vi "odometryfgv.vi"(7 "error in (no error)":errorcluster, 9 "wheelbase":dbl=250.0, 10 "Reset":bool) -> (0 "error out":errorcluster, 2 "XY Graph 2":cluster{"X":dbl, "Y":dbl}[](graph), 3 "X, Y, BEARING":cluster{dbl, dbl, dbl}={77.90712658947966, 981.2627307621673, -194.46797875856427})   [LabVIEW 2017]
uses:
  <vilib>/myRIO/Common/Instrument Driver Framework/myRIO v1.0/Encoder/typedefs/Encoder Signal Mode.ctl
  <vilib>/myRIO/Instrument Drivers/Onboard IO/Encoder/typedefs/Encoder Reference.ctl
  <vilib>/myRIO/Common/Instrument Driver Framework/Utilities/typedefs/myRIO Generic Hardware Reference.ctl
  <vilib>/myRIO/Common/Instrument Driver Framework/Utilities/typedefs/Hardware Version Enum.ctl
  <vilib>/myRIO/Common/Instrument Driver Framework/Utilities/typedefs/myRIO v1.0 Reference.ctl
  <vilib>/myRIO/Common/Instrument Driver Framework/Utilities/typedefs/Generic FPGA Reference.ctl
  <vilib>/myRIO/Common/Instrument Driver Framework/myRIO v1.0/Encoder/typedefs/Encoder Channels Enum.ctl
  <vilib>/myRIO/Common/Instrument Driver Framework/myRIO v1.0/Encoder/typedefs/Encoder Configuration v1.0.ctl
  <vilib>/userdefined/High Color/nirio_resource_hc.ctl
  <vilib>/myRIO/Common/Instrument Driver Framework/Utilities/vis/Is FPGA Ref Available.vi
  <vilib>/myRIO/Common/Instrument Driver Framework/myRIO v1.0/Encoder/vis/myRIO v1.1 Open Encoder.vi
  <vilib>/myRIO/Instrument Drivers/Onboard IO/Encoder/vis/Read.vi
  <vilib>/myRIO/Common/Instrument Driver Framework/Utilities/vis/Validate Channels.vi
  <vilib>/myRIO/Common/Instrument Driver Framework/myRIO v1.0/Encoder/vis/myRIO v1.0 Reserve Encoder.vi
  <vilib>/myRIO/Common/Instrument Driver Framework/myRIO v1.0/Encoder/vis/myRIO v1.0 Build MUX Configuration Encoder.vi
  <vilib>/myRIO/Common/Instrument Driver Framework/myRIO v1.0/Resource Manager/vis/myRIO v1.0 Reserve Channel List.vi
  <vilib>/myRIO/Common/Instrument Driver Framework/myRIO v1.0/Resource Manager/vis/myRIO v1.0 Create Configuration List.vi
  <vilib>/myRIO/Common/Instrument Driver Framework/myRIO v1.0/Resource Manager/vis/myRIO v1.0 Reserve Channel.vi
  <vilib>/myRIO/Common/Instrument Driver Framework/myRIO v1.0/Resource Manager/vis/myRIO v1.0 Unreserve Channel.vi
  <vilib>/myRIO/Common/Instrument Driver Framework/myRIO v1.0/Resource Manager/vis/myRIO v1.0 Build Mutex Name.vi
  <vilib>/Utility/VariantDataType/GetNumericInfo.vi
  <vilib>/Utility/error.llb/Error Cluster From Error Code.vi
  <vilib>/myRIO/Common/Instrument Driver Framework/myRIO v1.0/myRIO v1.1 Open.vi
  <vilib>/myRIO/Common/Instrument Driver Framework/Utilities/vis/IO Manager.vi
  <vilib>/myRIO/Common/Instrument Driver Framework/Utilities/vis/Configuration Manager.vi
  <vilib>/myRIO/Common/Instrument Driver Framework/myRIO v1.0/Resource Manager/vis/myRIO v1.0 Configure IO.vi
  <vilib>/myRIO/Common/Instrument Driver Framework/myRIO v1.0/myRIO v1.0 Close.vi
  <vilib>/myRIO/Common/Instrument Driver Framework/myRIO v1.0/Encoder/vis/myRIO v1.0 Configure Encoder.vi
  <vilib>/myRIO/Common/Instrument Driver Framework/myRIO v1.0/Encoder/vis/myRIO v1.0 Read Encoder.vi
  <vilib>/myRIO/Express VI/Onboard IO/Encoder/Encoder Express VI.xnode
  <vilib>/myRIO/Instrument Drivers/Onboard IO/Encoder/vis/myRIO Encoder Open.xnode
  <vilib>/myRIO/Instrument Drivers/Onboard IO/Encoder/Encoder.lvlib
panel:
  out "Waveform Chart":cluster{dbl, dbl, dbl}(graph)
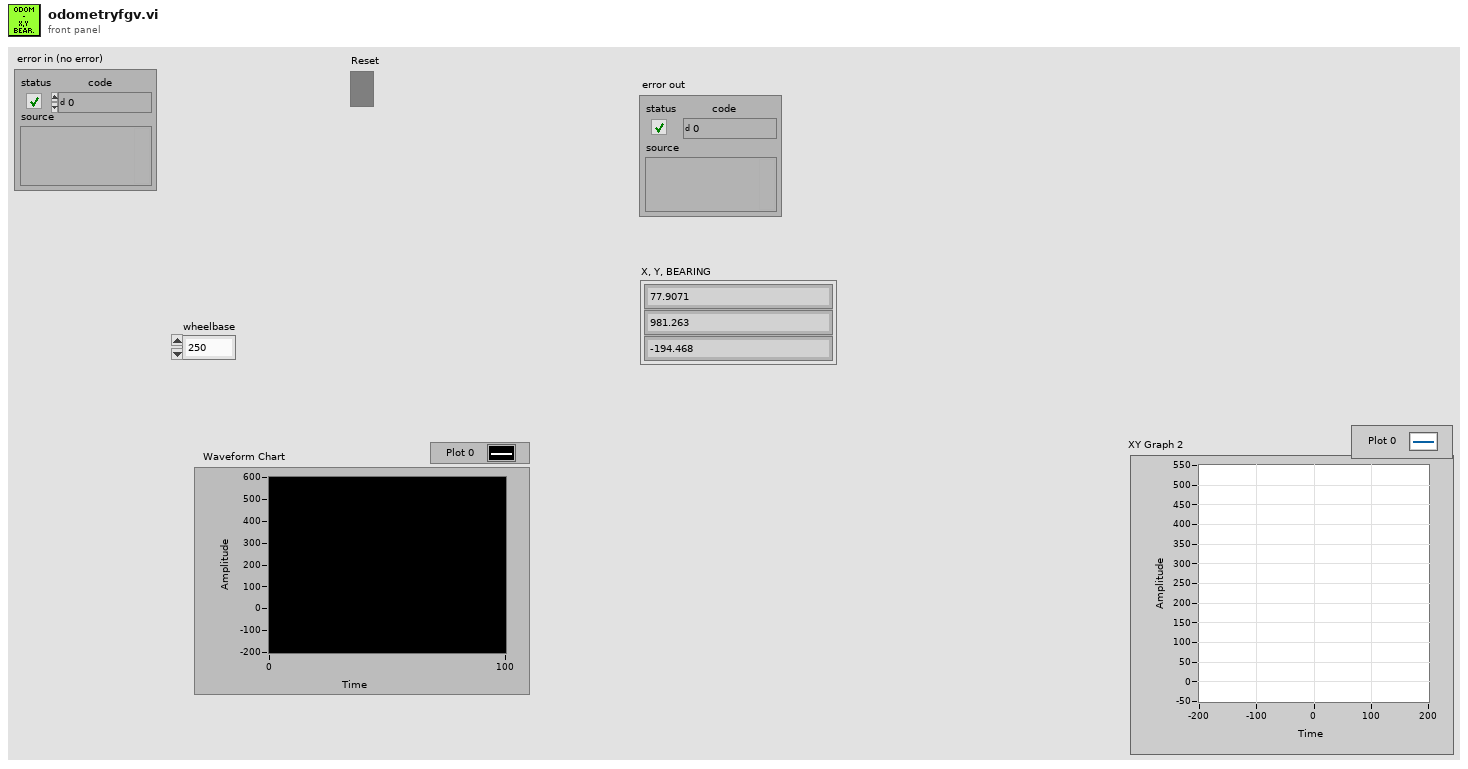
[diagram p1: front panel]
types:
  T1 = typedef "Encoder.lvlib/Encoder Reference.ctl" = cluster{"myRIO Reference":T2, "Encoder Channels Enum":T6}
  T2 = typedef "myRIO Generic Hardware Reference.ctl" = cluster{"myRIO Model":T3, "myRIO Hardware Reference":T4}
  T3 = typedef "Hardware Version Enum.ctl" = enum16{"Unknown", "myRIO-1900", "myRIO-1950", "roboRIO", "NI ELVIS RIO CM"}
  T4 = typedef "myRIO v1.0 Reference.ctl" = cluster{"Generic FPGA Reference":T5, "Allow multiple opens":bool}
  T5 = typedef "Generic FPGA Reference.ctl" = refnum<k20>
  T6 = typedef "Encoder Channels Enum.ctl" = enum16{"Not Connected", "C/ENC0", "C/ENC1", "A/ENC", "B/ENC", "DIO/ENC0", "DIO/ENC1", "DIO/ENC2", "DIO/ENC3", "DIO/ENC4"}
  T7 = typedef "Encoder Signal Mode.ctl" = enum16{"Quadrature phase signal", "Step and direction signal"}
  T8 = typedef "nirio_resource_hc.ctl" = tag
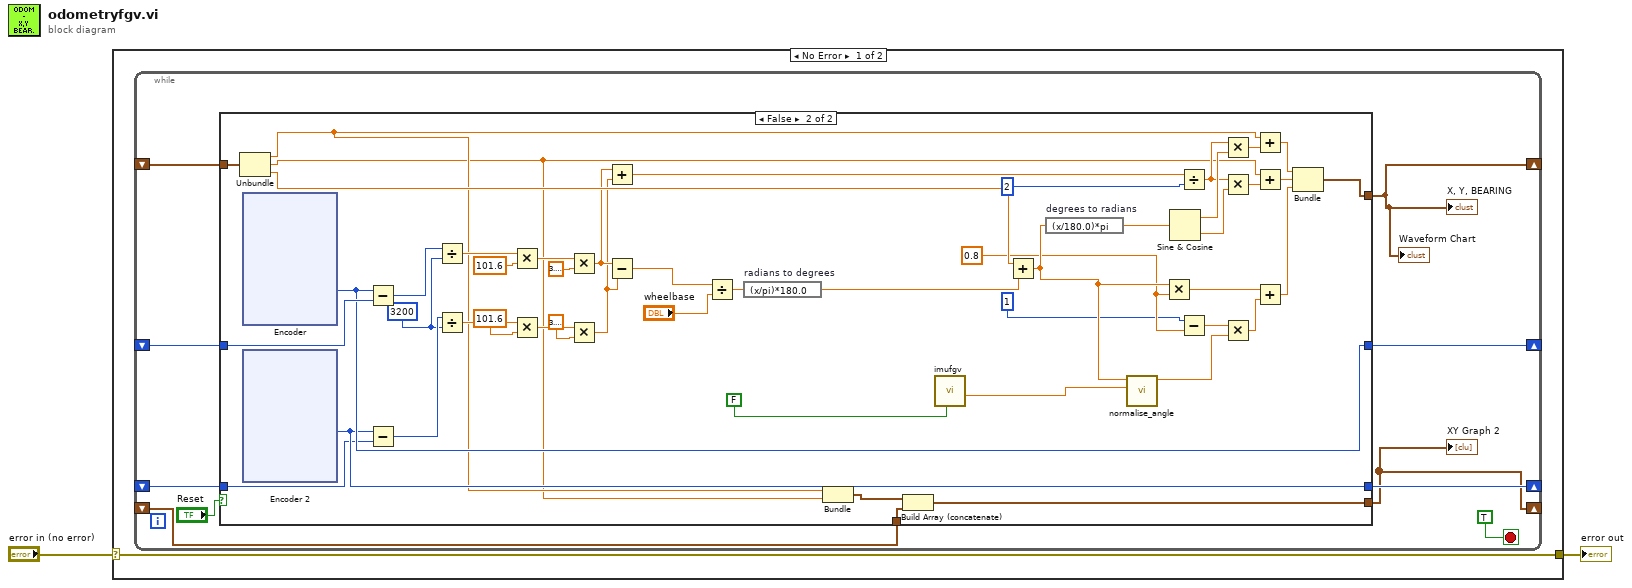
[diagram p0: block diagram]
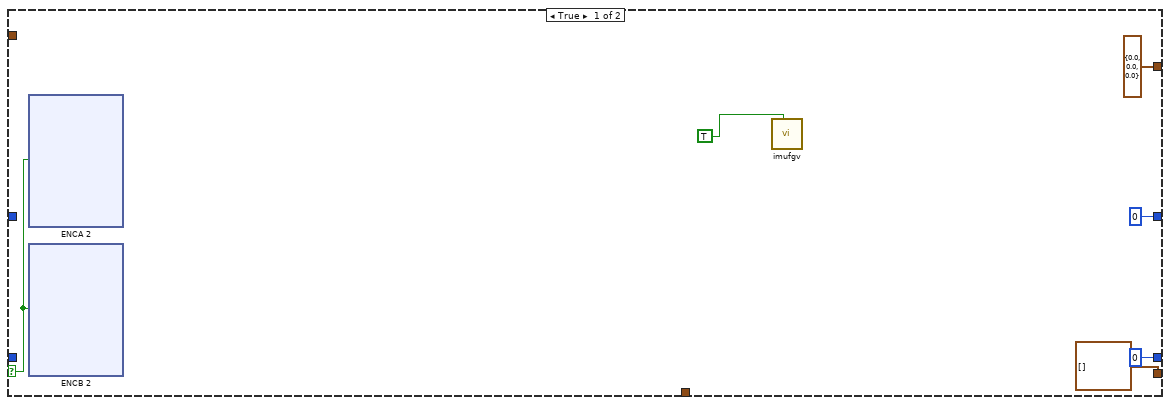
[diagram p2: hidden frame]
diagram:
  n1 = case shown="No Error" "error in (no error)" {
    selector: "error in (no error)" -> [w3 w253]
    tunnel: [w3 w253] -> w1
    frame No Error {
      n2 = while {
        shift-right: [w6] -> _
        shift-left: _ -> [w13]
        shift-right: [w11] -> _
        shift-left: _ -> [w10]
        shift-right: [w9] -> _
        shift-left: _ -> [w8]
        shift-right: [w4] -> _
        shift-left: _ -> [w5]
        stop <- TRUE stop-if-true
        n3 = case shown="False" "Reset" {
          selector: "Reset" -> [w16 _]
          tunnel: w13 -> [_ w160]
          tunnel: [cluster{dbl, dbl, dbl} {0.0, 0.0, 0.0} w118] -> w6
          tunnel: w10 -> [_ w149]
          tunnel: [0 w131] -> w11
          tunnel: [0 w130] -> w9
          tunnel: w8 -> [_ w129]
          tunnel: [cluster{dbl, dbl}[] [] w113] -> w4
          tunnel: w5 -> [_ w112]
          frame True {
            n4 = xnode "ENCA 2"("Reset Counter"=w16) -> ()  [unwired: 1 in, 4 out]
            n5 = xnode "ENCB 2"("Reset Counter"=w16) -> ()  [unwired: 1 in, 4 out]
            n6 = call "imufgv.vi"("Rset"=TRUE) -> ()  [unwired: 9 in, 2 out]
          }
          frame False {
            w122 = 0.8
            w144 = 3200
            n7 = Unbundle(w160) -> (w116:dbl, w115:dbl, w156:dbl)
            n8 = xnode "Encoder"() -> ("Counter Value"=w131:i32)  [unwired: 2 in, 3 out]
            n9 = xnode "Encoder 2"() -> ("Counter Value"=w130:i32)  [unwired: 2 in, 3 out]
            n10 = Subtract(x=w131, y=w149) -> (x-y=w146:i32)
            n11 = Subtract(x=w130, y=w129) -> (x-y=w145:i32)
            n12 = Divide(x=w146, y=w144) -> (x/y=w143:dbl)
            n13 = Divide(x=w145, y=w144) -> (x/y=w135:dbl)
            n14 = Multiply(x=w143, y=101.6) -> (x*y=w142:dbl)
            n15 = Multiply(x=w135, y=101.6) -> (x*y=w137:dbl)
            n16 = Multiply(x=w142, y=3.141592653589793) -> (x*y=w141:dbl)
            n17 = Multiply(x=w137, y=3.141592653589793) -> (x*y=w136:dbl)
            n18 = Add(x=w141, y=w136) -> (x+y=w147:dbl)
            n19 = Subtract(x=w141, y=w136) -> (x-y=w148:dbl)
            n20 = Divide(x=w148, y="wheelbase") -> (x/y=w157:dbl)
            n21 = expression code="(x/pi)*180.0" "radians to degrees"(w157) -> (w127:dbl)
            n22 = Bundle(w116, w115) -> (w114:cluster{dbl, dbl})  [unwired: 1 in]
            n23 = Build Array (concatenate)(w114, w112) -> (w113:cluster{dbl, dbl}[])
            n24 = call "imufgv.vi"("Rset"=FALSE) -> ("yaw"=w126:dbl)  [unwired: 9 in, 1 out]
            n25 = Add(x=w156, y=w127) -> (x+y=w123:dbl)
            n26 = expression code="(x/180.0)*pi" "degrees to radians"(w123) -> (w155:dbl)
            n27 = call "normalise_angle.vi"("target -180 .. 180"=w126, "current"=w123) -> ("travel_direction"=w124:dbl)  [unwired: 9 in]
            n28 = Multiply(x=w123, y=w122) -> (x*y=w121:dbl)
            n29 = Sine & Cosine(0:w155) -> (1:w154:dbl, 2:w153:dbl)
            n30 = Divide(x=w147, y=2) -> (x/y=w150:dbl)
            n31 = Subtract(x=1, y=w122) -> (x-y=w125:dbl)
            n32 = Multiply(x=w150, y=w154) -> (x*y=w151:dbl)
            n33 = Multiply(x=w150, y=w153) -> (x*y=w152:dbl)
            n34 = Multiply(x=w125, y=w124) -> (x*y=w120:dbl)
            n35 = Add(x=w116, y=w151) -> (x+y=w133:dbl)
            n36 = Add(x=w115, y=w152) -> (x+y=w132:dbl)
            n37 = Add(x=w121, y=w120) -> (x+y=w119:dbl)
            n38 = Bundle(w133, w132, w119) -> (w118:cluster{dbl, dbl, dbl})  [unwired: 1 in]
          }
        }
        "X, Y, BEARING" <- w6
        "Waveform Chart" <- w6
        "XY Graph 2" <- w4
      }
    }
    frame Error {
    }
  }
  "error out" <- w1
